vi "FTW-URI-FromFilepath.vi"(0 "Path":path, 11 "error in":errorcluster) -> (4 "URI":string, 15 "error out":errorcluster)   [LabVIEW 2013]
panel:
  # "Inputs"
  # "Outputs"
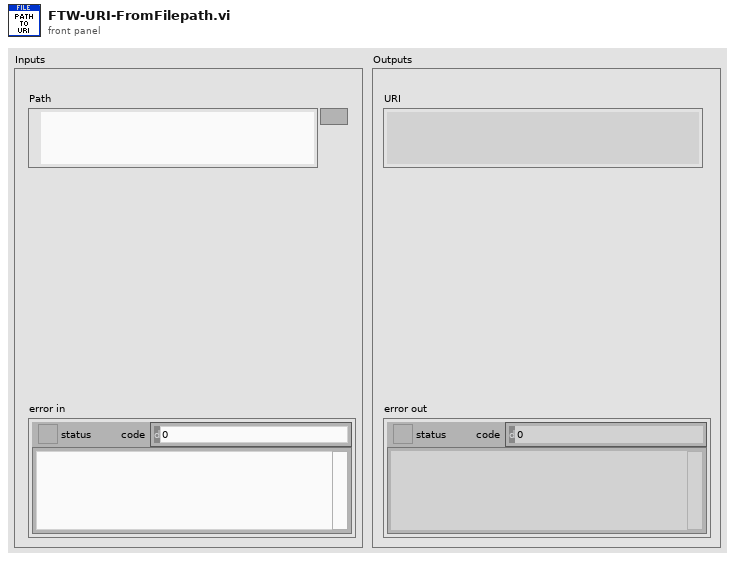
[diagram p1: front panel]
types:
  T1 = enum32{"invalid OS target", "Mac OS", "Windows 3.1", "Windows 95/NT", "Solaris 1", "Solaris 2", "HP-UX", "PowerMAX", "Linux", "Irix", "Rhapsody", "BeOS", "AIX", "OSF1", "VxWorks", "PharLap", "Carbon", "RTX", "Windows x64", "Linux x64"}
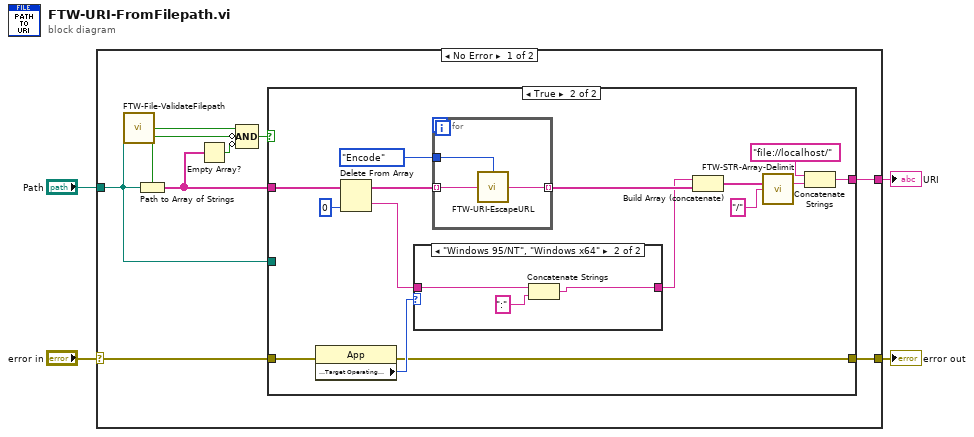
[diagram p0: block diagram]
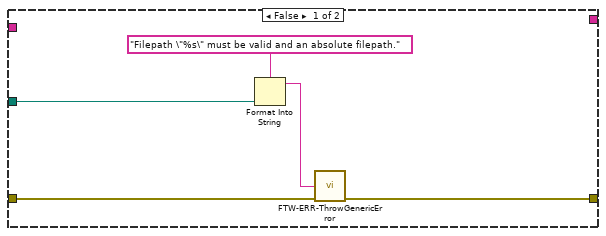
[diagram p2: hidden frame]
diagram:
  n1 = case shown="No Error" "error in" {
    selector: "error in" -> [w8 w41]
    tunnel: [w9 _] -> w4
    tunnel: "Path" -> [w5 _]
    tunnel: [w7 w41] -> w1
    frame No Error {
      n2 = call "FTW-File-ValidateFilepath.vi"("Filepath"=w5) -> ("Valid?"=w10:bool)
      n3 = Path to Array of Strings(0:w5) -> (1:w11:bool, 2:w13:string[])
      n4 = Empty Array?(array=w13) -> (empty?=w12:bool)
      n5 = Compound Arithmetic op=AND(w10, invert w11, invert w12) -> (w6:bool)
      n6 = case shown="True" w6 {
        tunnel: w13 -> [_ w26]
        tunnel: [_ w22] -> w9
        tunnel: w8 -> [w18 w21]
        tunnel: [w17 w20] -> w7
        tunnel: w5 -> [w16 _]
        frame False {
          n7 = Format Into String(format string="Filepath \"%s\" must be valid and an absolute filepath." ("Error Message"), w16) -> (resulting string=w14:string)  [unwired: 2 in, 1 out]
          n8 = call "FTW-ERR-ThrowGenericError.vi"("Error Message"=w14, "error in"=w18) -> ("error out"=w17:errorcluster)  [unwired: 13 in]
        }
        frame True {
          n9 = property class="App"(error in=w21) -> (error out=w20:errorcluster, "Application:Target Operating System"=w29:T1)  [unwired: 1 in, 1 out]
          n10 = Delete From Array(array=w26, index=0) -> (deleted portion=w30:string, array with subset deleted=w27:string[])  [unwired: 1 in]
          n11 = case shown="\"Windows 95/NT\", \"Windows x64\"" w29 {
            tunnel: w30 -> [w34 w37]
            tunnel: [w34 w35] -> w31
            frame Default {
            }
            frame "Windows 95/NT", "Windows x64" {
              n12 = Concatenate Strings(w37, ":" ("string")) -> (w35:string)
            }
          }
          n13 = for {
            tunnel: w27 -> [w40] mode=indexing
            tunnel: [w39] -> w33 mode=indexing
            tunnel: enum16{"Encode", "Decode"}."Encode" ("Direction") -> [w38]
            n14 = call "FTW-URI-EscapeURL.vi"("Input"=w40, "Direction"=w38) -> ("Output"=w39:string)
          }
          n15 = Build Array (concatenate)(w31, w33) -> (w32:string[])
          n16 = call "FTW-STR-Array-Delimit.vi"("Array of Strings"=w32, "Delimiter"="/") -> ("Delimited String"=w25:string)  [unwired: 13 in]
          n17 = Concatenate Strings("file://localhost/", w25) -> (w22:string)
        }
      }
    }
    frame Error {
    }
  }
  "error out" <- w1
  "URI" <- w4
